vi "Save 1D array.vi"(0 "ÆT":dbl format="%.2e", 1 "Data":dbl[](array[numeric]) format="%.2e", 2 "File Path":path) -> ()   [LabVIEW 2024]
panel:
  out "Error Code":i32
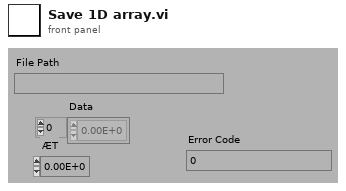
[diagram p1: front panel]
types:
  T1 = enum16{"open", "replace", "create", "open or create", "replace or create", "replace or create with confirmation"}
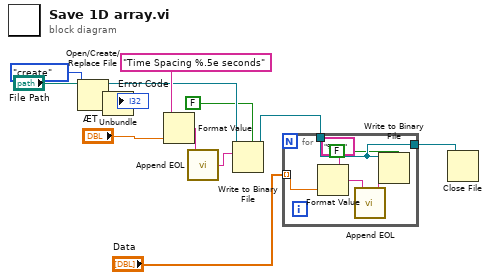
[diagram p0: block diagram]
diagram:
  n1 = Open/Create/Replace File(file path (use dialog)="File Path", operation (0:open)=T1."create") -> (refnum out=w8:refnum<file>, error out=w4:errorcluster)  [unwired: 4 in, 1 out]
  n2 = Unbundle(w4) -> ("code"=→"Error Code":i32)  [unwired: 2 out]
  n3 = Format Value(format string="Time Spacing %.5e seconds", value (0)="ÆT") -> (output string=w10:string)  [unwired: 1 in]
  n4 = call "Append EOL.vi"("INPUT STRING"=w10) -> ("OUTPUT STRING (PLUS End of Line)"=w9:string)
  n5 = Write to Binary File(file (use dialog)=w8, data=w9, 5:FALSE ("prepend array or string size? (T)")) -> (refnum out=w6:refnum<file>)  [unwired: 3 in, 2 out]
  n6 = for {
    tunnel: "Data" -> [w19] mode=indexing
    tunnel: w6 -> [w15]
    tunnel: [w15] -> w5
    n7 = Format Value(format string="%.8e", value (0)=w19) -> (output string=w17:string)  [unwired: 1 in]
    n8 = call "Append EOL.vi"("INPUT STRING"=w17) -> ("OUTPUT STRING (PLUS End of Line)"=w16:string)
    n9 = Write to Binary File(file (use dialog)=w15, data=w16, 5:FALSE ("prepend array or string size? (T)")) -> ()  [unwired: 3 in, 3 out]
  }
  n10 = Close File(refnum=w5) -> ()  [unwired: 1 in, 2 out]
